vi "Status ProgramState.vi"(8 "error in (no error)":errorcluster, 10 "Address (0)":i32, 11 "VISA resource name":refnum<visa-resource-name>) -> (0 "error out":errorcluster, 2 "Program State":T1 {"remaining time" format="%<%H:%M>t"}, 3 "VISA resource name out":refnum<visa-resource-name>)   [LabVIEW 2016, in "Environment Chamber.lvlib" / "Climatic Chamber.lvlib"]
doc: "<b>Program execution monitor</B>\n\nReturns the operation state parameter when a program is operating."
uses:
  Climatic Chamber.lvlib
  Private/Type Defs/Program OpState Cluster.ctl
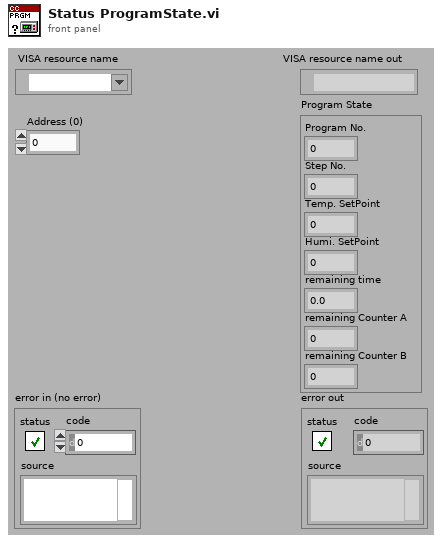
[diagram p1: front panel]
types:
  T1 = typedef "Environment Chamber.lvlib/Climatic Chamber.lvlib/Program OpState Cluster.ctl" = cluster{"Program No.":i32, "Step No.":i32, "Temp. SetPoint":dbl, "Humi. SetPoint":dbl, "remaining time":dbl, "remaining Counter A":i32, "remaining Counter B":i32}
  T2 = cluster{i32, i32, "output 1":dbl, "output 1":dbl, dbl, i32, i32}
  T3 = cluster{i32, i32, "default value 1":dbl, "default value 1":dbl, dbl, i32, i32}
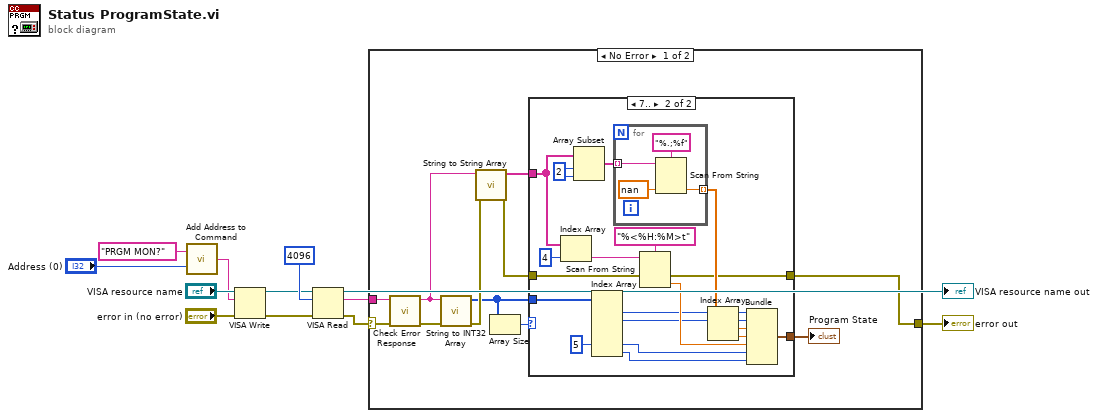
[diagram p0: block diagram]
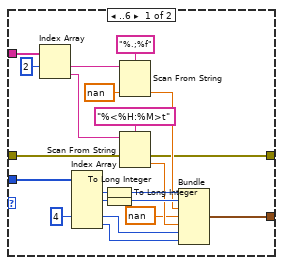
[diagram p2: hidden frame]
diagram:
  n1 = call "Add Address to Command.vi"("Address (0)"="Address (0)", "Command"="PRGM MON?") -> ("Command OUT"=w5:string)
  n2 = VISA Write(VISA resource name="VISA resource name", write buffer=w5, error in (no error)="error in (no error)") -> (VISA resource name out=w9:refnum<visa-resource-name>, error out=w8:errorcluster)  [unwired: 1 out]
  n3 = VISA Read(VISA resource name=w9, byte count=u32 4096, error in (no error)=w8) -> (VISA resource name out=→"VISA resource name out":refnum<visa-resource-name>, read buffer=w3:string, error out=w4:errorcluster)  [unwired: 1 out]
  n4 = case shown="No Error" w4 {
    selector: w4 -> [w20 w68]
    tunnel: w3 -> [w21 _]
    tunnel: [w15 w68] -> w2
    frame No Error {
      n5 = call "Check Error Response.vi"("error in (no error)"=w20, "read String"=w21) -> ("error out"=w22:errorcluster, "String out"=w13:string)  [unwired: 7 in, 1 out]
      n6 = call "String to INT32 Array.vi"("error in (no error)"=w22, "String received"=w13) -> ("error out"=w23:errorcluster, "Array Data"=w18:i32[])  [unwired: 8 in]
      n7 = call "String to String Array.vi"("error in (no error)"=w23, "String received"=w13) -> ("error out"=w16:errorcluster, "Array Data"=w17:string[])  [unwired: 8 in]
      n8 = Array Size(array=w18) -> (size(s)=w19:i32)
      n9 = case shown="7.." w19 {
        tunnel: w18 -> [w44 w63]
        tunnel: w17 -> [w37 w51]
        tunnel: w16 -> [w36 w56]
        tunnel: [w24 w45] -> w15
        tunnel: [w30 w54] -> w14
        frame ..6 {
          n10 = Index Array(array=w37, index #1=2 ("index")) -> (element #1=w28:string, element #2=w29:string)  [unwired: 1 in]
          n11 = Index Array(array=w44, index #4=4 ("index")) -> (element #1=w43:i32, element #2=w42:i32, element #4=w34:i32, element #5=w33:i32)  [unwired: 4 in, 1 out]
          n12 = To Long Integer(number=w43) -> (32bit integer=w41:i32)
          n13 = To Long Integer(number=w42) -> (32bit integer=w40:i32)
          n14 = Scan From String(format string="%.;%f", input string=w28, default 1=nan ("output 1")) -> (output 1=w25:dbl)  [unwired: 2 in, 3 out]
          n15 = Scan From String(format string="%<%H:%M>t", input string=w29, error in=w36) -> (error out=w24:errorcluster, output 1=w32:dbl)  [unwired: 2 in, 2 out]
          n16 = Bundle(w41, w40, "output 1"=w25, "output 1"=nan, w32, w34, w33) -> (w30:T2)  [unwired: 1 in]
        }
        frame 7.. {
          w50 = 2 ("index")
          n17 = Index Array(array=w51, index=4) -> (element=w58:string)
          n18 = Array Subset(array=w51, index=w50, length=w50) -> (w49:string[])
          n19 = Index Array(array=w63, index #5=5 ("index")) -> (element #1=w53:i32, element #2=w52:i32, element #5=w61:i32, element #6=w60:i32)  [unwired: 5 in, 2 out]
          n20 = for {
            tunnel: w49 -> [w67] mode=indexing
            tunnel: [w64] -> w46 mode=indexing
            n21 = Scan From String(format string="%.;%f", input string=w67, default 1=nan ("default value 1")) -> (output 1=w64:dbl)  [unwired: 2 in, 3 out]
          }
          n22 = Scan From String(format string="%<%H:%M>t", input string=w58, error in=w56) -> (error out=w45:errorcluster, output 1=w55:dbl)  [unwired: 2 in, 2 out]
          n23 = Index Array(array=w46) -> (element #1=w48:dbl, element #2=w47:dbl)  [unwired: 2 in]
          n24 = Bundle(w53, w52, "default value 1"=w48, "default value 1"=w47, w55, w61, w60) -> (w54:T3)  [unwired: 1 in]
        }
      }
      "Program State" <- w14
    }
    frame Error {
    }
  }
  "error out" <- w2
